vi "Get Item Resource.vi"(8 "error in (no error)":errorcluster, 10 "ItemName":string, 11 "GObject in":refnum<class "GObject.lvclass">) -> (0 "error out":errorcluster, 1 "Found?":bool, 2 "Resource":T2, 3 "GObject out":refnum<class "GObject.lvclass">, 5 "Languages":T1[](array[typedef]))   [LabVIEW 2013, in "SET Project Data.lvlib" / "GObject.lvclass"]
uses:
  GObject.lvclass
  Types/ProjFile_Resource Entry.ctl
  Types/ProjFile_Language Entry.ctl
  GObject.lvclass/GObject.ctl
  Resource Data Class/Resource Data.lvclass/Resource Data.ctl
  Resource Data Class/Read Languages.vi
  Resource Data Class/Resource Data.lvclass
  SET Project Data.lvlib
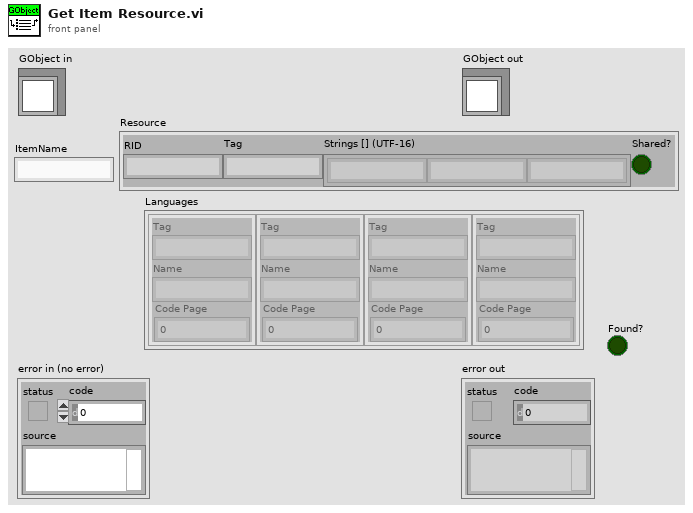
[diagram p1: front panel]
types:
  T1 = typedef "SET Project Data.lvlib/ProjFile_Language Entry.ctl" = cluster{"Tag":string, "Name":string, "Code Page":u16}
  T2 = typedef "SET Project Data.lvlib/ProjFile_Resource Entry.ctl" = cluster{"RID":string, "Tag":string, "Strings [] (UTF-16)":string[], "Shared?":bool}
  T3 = typedef "SET Project Data.lvlib/ProjFile_Language Data.ctl" = cluster{"Tag":string, "Name":string, "Code Page":u16}
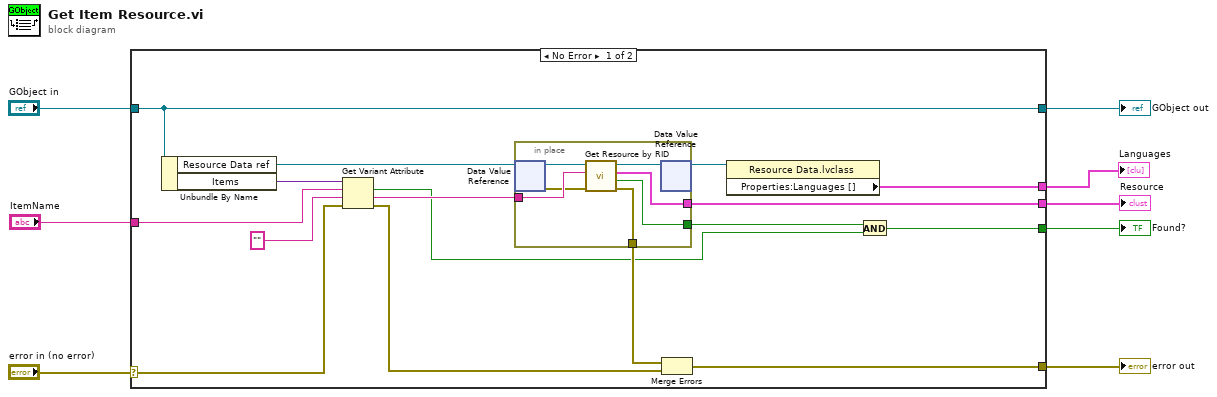
[diagram p0: block diagram]
diagram:
  n1 = case shown="No Error" "error in (no error)" {
    selector: "error in (no error)" -> [w21 w33]
    tunnel: [w16 w33] -> w7
    tunnel: [w24 w32] -> w5
    tunnel: "GObject in" -> [w24 w32]
    tunnel: "ItemName" -> [w22 _]
    tunnel: [w15 _] -> w2
    tunnel: [w12 _] -> w3
    tunnel: [w10 _] -> w1
    frame No Error {
      n2 = Unbundle By Name(w24) -> ("Resource Data ref"=w20:refnum<data-value>, "Items"=w23:variant)
      n3 = Get Variant Attribute(Variant=w23, name=w22, default value (empty Variant)="", error in=w21) -> (found=w13:bool, value=w19:string, error out=w18:errorcluster)  [unwired: 1 out]
      n4 = in-place {
        in-place-border: w19 -> [w29]
        in-place-border: [w28] -> w14
        in-place-border: [w25] -> w17
        in-place-border: [w27] -> w15
        n5 = in-place-dvr #1(w20) -> (w31:refnum<class "Resource Data.lvclass">, w26:errorcluster)
        n6 = call "Get Resource by RID.vi"("error in (no error)"=w26, "RID"=w29, "LangFile in"=w31) -> ("error out"=w25:errorcluster, "Found?"=w28:bool, "Resource"=w27:T2, "LangFile out"=w30:refnum<class "Resource Data.lvclass">)  [unwired: 4 in, 1 out]
        n7 = in-place-dvr #1(w30) -> (w11:refnum<data-value>)  [unwired: 1 out]
      }
      n8 = Merge Errors(w17, w18) -> (w16:errorcluster)
      n9 = property class="Resource Data.lvclass"(reference=w11) -> ("Properties:Languages []"=w10:T3[])  [unwired: 1 in, 2 out]
      n10 = And(x=w14, y=w13) -> (x .and. y?=w12:bool)
    }
    frame Error {
    }
  }
  "error out" <- w7
  "GObject out" <- w5
  "Found?" <- w3
  "Resource" <- w2
  "Languages" <- w1
